vi "GetReadVITemplatePath.vi"(7 "Include error terminals":bool, 8 "error in (no error)":errorcluster, 11 "MultiDimArrElemScripter in":refnum<class "MultiDimArrElemScripter.lvclass">) -> (0 "error out":errorcluster, 2 "VI Path":path, 3 "MultiDimArrElemScripter out":refnum<class "MultiDimArrElemScripter.lvclass">)   [LabVIEW 2021, in "MemberVICreation.lvlib" / "MultiDimArrElemScripter.lvclass"]
uses:
  <resource>/Framework/Providers/LVClassLibrary/NewAccessors/MultiDimArrElemScripter/MultiDimArrElemScripter.lvclass
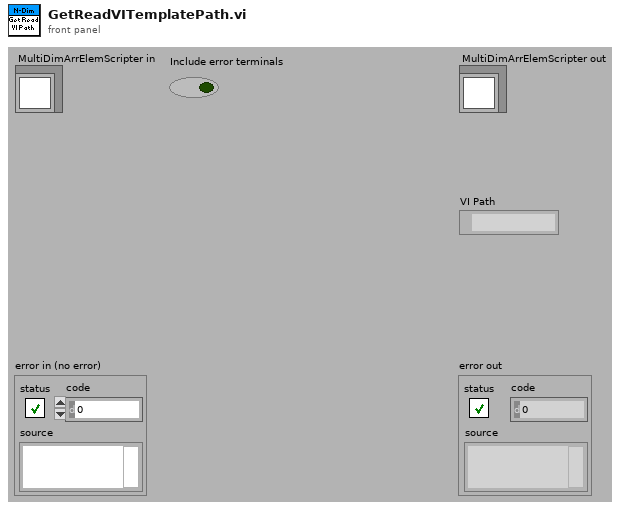
[diagram p1: front panel]
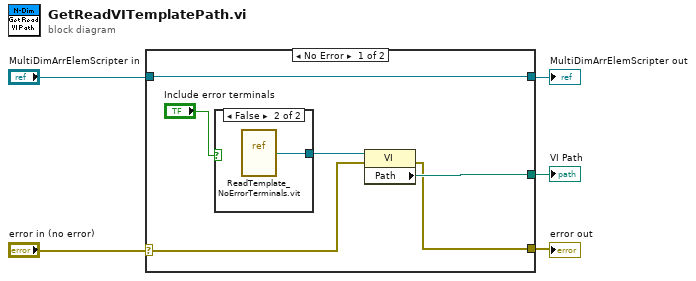
[diagram p0: block diagram]
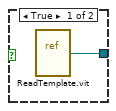
[diagram p2: hidden frame]
diagram:
  n1 = case shown="No Error" "error in (no error)" {
    selector: "error in (no error)" -> [w8 w15]
    tunnel: [w7 w15] -> w2
    tunnel: [w11 w14] -> w5
    tunnel: "MultiDimArrElemScripter in" -> [w11 w14]
    tunnel: [w9 _] -> w1
    frame No Error {
      n2 = case shown="False" "Include error terminals" {
        tunnel: [w12 w13] -> w10
        frame True {
          n3 = vi-ref <resource>:"ReadTemplate.vit"() -> (w12:refnum<vi>)
        }
        frame False {
          n4 = vi-ref <resource>:"ReadTemplate_NoErrorTerminals.vit"() -> (w13:refnum<vi>)
        }
      }
      n5 = property class="VI"(reference=w10, error in=w8) -> (error out=w7:errorcluster, "Path"=w9:path)  [unwired: 1 out]
    }
    frame Error {
    }
  }
  "error out" <- w2
  "VI Path" <- w1
  "MultiDimArrElemScripter out" <- w5
